vi "查找元素名称ByName.vi"(6 "offset (0)":i32 caption="偏移量(0)", 10 "Element Name":string caption="元素名", 11 "string":string caption="字符串") -> (1 "after substring":string caption="子字符串之后", 2 "match substring":string caption="匹配子字符串", 3 "before substring":string caption="子字符串之前", 4 "offset past match":i32 caption="匹配后偏移量")   [LabVIEW 2017]
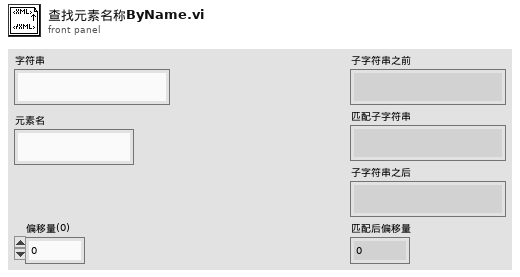
[diagram p1: front panel]
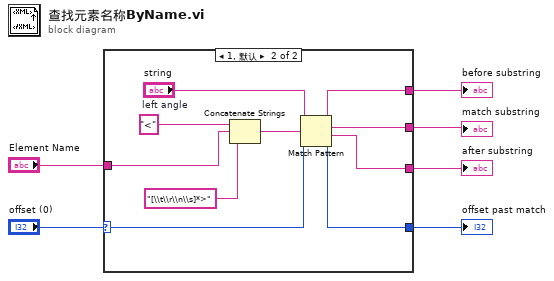
[diagram p0: block diagram]
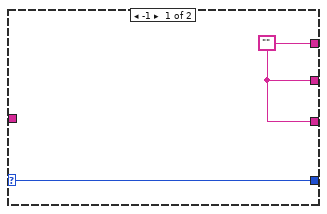
[diagram p2: hidden frame]
diagram:
  n1 = case shown="1, 默认" "offset (0)" {
    selector: "offset (0)" -> [w8 w11]
    tunnel: [w7 w15] -> w6
    tunnel: [w7 w14] -> w5
    tunnel: [w8 w13] -> w4
    tunnel: [w7 w12] -> w3
    tunnel: "Element Name" -> [_ w9]
    frame -1 {
      w7 = ""
    }
    frame 1, Default {
      w18 = "<"  # left angle
      n2 = Concatenate Strings(w18, w9, "[\\t\\r\\n\\s]*>" ("regular expression")) -> (w16:string)
      n3 = Match Pattern(string="string", regular expression=w16, offset (0)=w11) -> (before substring=w15:string, match substring=w12:string, after substring=w14:string, offset past match=w13:i32)
    }
  }
  "before substring" <- w6
  "match substring" <- w3
  "after substring" <- w5
  "offset past match" <- w4
